vi "Finish.vi"   [LabVIEW 2013]
doc: "This VI is called just before exiting. It is expected to close I/O refnum, save collected data, etc."
uses:
  <vilib>/Rock Robotics/WPI/RobotDrive/WPI_RobotDriveGetSetRefNum.vi
  <vilib>/Rock Robotics/WPI/Joystick/WPI_JoystickGetSetRefNum.vi
types:
  T1 = typedef "WPI_RobotDriveDevRef.ctl" = cluster{"DevStatus":errorcluster, "Motors[]":T2[], "Square Inputs":bool, "Max Output":dbl, "Isochronous":bool}
  T2 = typedef "WPI_MotorControlDeviceRef.ctl" = cluster{"DeviceStatus":errorcluster, "Type":enum16{"PWM", "CAN"}, "PWM":cluster{"Digital Module":T3, "PWM Channel":T4, "DeadBand":T5}, "CAN":cluster{"Device Number":u8, "Control Mode":T6, "Semaphore":T7, "Max Vout":dbl}, "Invert":bool, "TransformRef":T8, "InvTransformRef":T8}
  T3 = typedef "FPGA_TypedefDigitalModule.ctl" = enum16{"Digital Module 1", "Digital Module 2"}
  T4 = typedef "FPGA_DIOPWMChannel.ctl" = enum8{"PWM 1", "PWM 2", "PWM 3", "PWM 4", "PWM 5", "PWM 6", "PWM 7", "PWM 8", "PWM 9", "PWM 10", "Invalid"}
  T5 = typedef "WPI_PWMDeadband.ctl" = cluster{"Name":string, "maxPositivePwm":i32, "minPositivePwm":i32, "centerPwm":i32, "maxNegativePwm":i32, "minNegativePwm":i32, "angularRange":u16}
  T6 = typedef "WPI_CANJaguar_ControlMode.ctl" = enum8{"Percent VBus", "Current", "Speed", "Position", "Voltage"}
  T7 = typedef "Semaphore RefNum" = refnum<k1>
  T8 = typedef "WPI_PWMTransform_ConPane.ctl" = refnum<vi>
  T9 = typedef "WPI_JoystickDevRef.ctl" = cluster{"Device":T10}
  T10 = typedef "WPI_JoystickDeviceEnum.ctl" = enum16{"USB 1", "USB 2", "USB 3", "USB 4", "Kinect 1", "Kinect 2"}
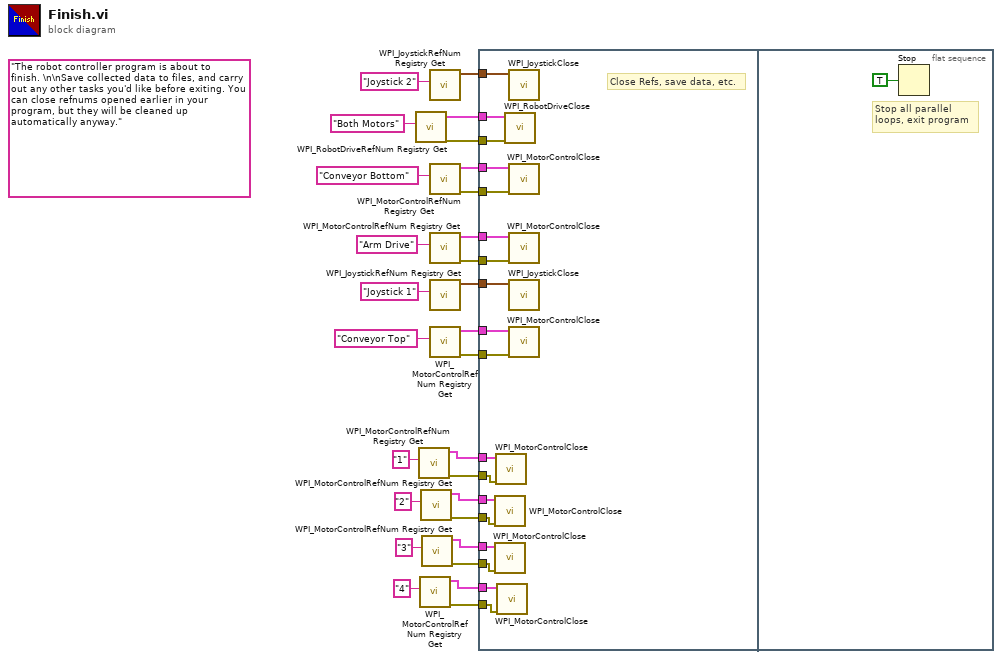
[diagram p0: block diagram]
diagram:
  (unwired) "The robot controller program is about to finish. \n\nSave collected data to files, and carry out any other tasks you'd like before exiting. You can close refnums opened earlier in your program, but they will be cleaned up automatically anyway."
  n1 = call <vilib>:"WPI_RobotDriveRefNum Registry Get.vi"("refnum name"="Both Motors") -> ("error out"=w13:errorcluster, "RobotDriveDevRef"=w14:T1)  [unwired: 1 in, 8 out]
  n2 = call <vilib>:"WPI_MotorControlRefNum Registry Get.vi"("refnum name"="1") -> ("error out"=w7:errorcluster, "MotorControlDevRef"=w8:T2)  [unwired: 9 in]
  n3 = call <vilib>:"WPI_MotorControlRefNum Registry Get.vi"("refnum name"="4") -> ("error out"=w1:errorcluster, "MotorControlDevRef"=w2:T2)  [unwired: 9 in]
  n4 = call <vilib>:"WPI_MotorControlRefNum Registry Get.vi"("refnum name"="2") -> ("error out"=w5:errorcluster, "MotorControlDevRef"=w6:T2)  [unwired: 9 in]
  n5 = call <vilib>:"WPI_MotorControlRefNum Registry Get.vi"("refnum name"="3") -> ("error out"=w3:errorcluster, "MotorControlDevRef"=w4:T2)  [unwired: 9 in]
  n6 = call <vilib>:"WPI_JoystickRefNum Registry Get.vi"("refnum name"="Joystick 2") -> ("JoystickDevRef"=w23:T9)  [unwired: 1 in, 9 out]
  n7 = call <vilib>:"WPI_MotorControlRefNum Registry Get.vi"("refnum name"="Conveyor Bottom") -> ("error out"=w18:errorcluster, "MotorControlDevRef"=w19:T2)  [unwired: 9 in]
  n8 = call <vilib>:"WPI_MotorControlRefNum Registry Get.vi"("refnum name"="Arm Drive") -> ("error out"=w25:errorcluster, "MotorControlDevRef"=w26:T2)  [unwired: 9 in]
  n9 = call <vilib>:"WPI_JoystickRefNum Registry Get.vi"("refnum name"="Joystick 1") -> ("JoystickDevRef"=w27:T9)  [unwired: 1 in, 9 out]
  n10 = call <vilib>:"WPI_MotorControlRefNum Registry Get.vi"("refnum name"="Conveyor Top") -> ("error out"=w20:errorcluster, "MotorControlDevRef"=w21:T2)  [unwired: 9 in]
  n11 = flat-sequence {
    tunnel: w27 -> [w46]
    tunnel: w26 -> [w45]
    tunnel: w25 -> [w44]
    tunnel: w23 -> [w43]
    tunnel: w21 -> [w42]
    tunnel: w20 -> [w41]
    tunnel: w19 -> [w40]
    tunnel: w18 -> [w39]
    tunnel: w14 -> [w38]
    tunnel: w13 -> [w37]
    tunnel: w8 -> [w36]
    tunnel: w7 -> [w35]
    tunnel: w6 -> [w34]
    tunnel: w5 -> [w33]
    tunnel: w4 -> [w32]
    tunnel: w3 -> [w31]
    tunnel: w2 -> [w30]
    tunnel: w1 -> [w29]
    frame #0 {
      # "Close Refs, save data, etc."
      n12 = call <vilib>:"WPI_MotorControlClose.vi"("error in (no error)"=w33, "MotorControlDevRef"=w34) -> ()  [unwired: 9 in, 1 out]
      n13 = call <vilib>:"WPI_MotorControlClose.vi"("error in (no error)"=w31, "MotorControlDevRef"=w32) -> ()  [unwired: 9 in, 1 out]
      n14 = call <vilib>:"WPI_MotorControlClose.vi"("error in (no error)"=w35, "MotorControlDevRef"=w36) -> ()  [unwired: 9 in, 1 out]
      n15 = call <vilib>:"WPI_MotorControlClose.vi"("error in (no error)"=w29, "MotorControlDevRef"=w30) -> ()  [unwired: 9 in, 1 out]
      n16 = call <vilib>:"WPI_RobotDriveClose.vi"("error in (no error)"=w37, "RobotDriveDevRef"=w38) -> ()  [unwired: 10 out]
      n17 = call <vilib>:"WPI_JoystickClose.vi"("JoystickDevRef"=w43) -> ()  [unwired: 11 out]
      n18 = call <vilib>:"WPI_MotorControlClose.vi"("error in (no error)"=w39, "MotorControlDevRef"=w40) -> ()  [unwired: 9 in, 1 out]
      n19 = call <vilib>:"WPI_MotorControlClose.vi"("error in (no error)"=w44, "MotorControlDevRef"=w45) -> ()  [unwired: 9 in, 1 out]
      n20 = call <vilib>:"WPI_JoystickClose.vi"("JoystickDevRef"=w46) -> ()  [unwired: 11 out]
      n21 = call <vilib>:"WPI_MotorControlClose.vi"("error in (no error)"=w41, "MotorControlDevRef"=w42) -> ()  [unwired: 9 in, 1 out]
    }
    frame #1 {
      # "Stop all parallel\nloops, exit program"
      n22 = Stop(stop? (T)=TRUE ("Quit")) -> ()
    }
  }
